vi "JSON Array To LV Enum.vi"(7 "Name Override":string, 8 "Error In":errorcluster, 10 "JSON Array":string, 11 "Enum Dest Dir":path) -> (0 "Error Out":errorcluster)   [LabVIEW 2011, in "LMH-Toolbox.lvlib" / "LMH-Scripting.lvlib"]
doc: "Script a typedef enum control from a JSON array."
uses:
  LMH-Scripting.lvlib
  <vilib>/Utility/miscctls.llb/LVPointTypeDef.ctl
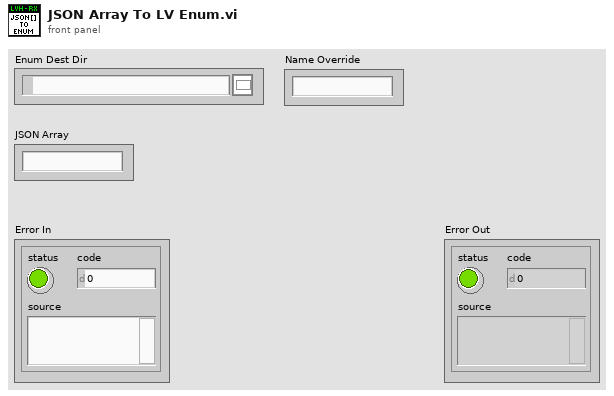
[diagram p1: front panel]
types:
  T1 = enum32{"not a control VI", "control", "typedef", "strict typedef"}
  T2 = typedef "LVPointTypeDef.ctl" = cluster{"Horizontal":i16, "Vertical":i16}
  T3 = enum32{"invalid VI type", "Standard VI", "Control VI", "Global VI", "Polymorphic VI", "Configuration VI", "SubSystem", "Facade VI", "Method VI", "Statechart Diagram VI"}
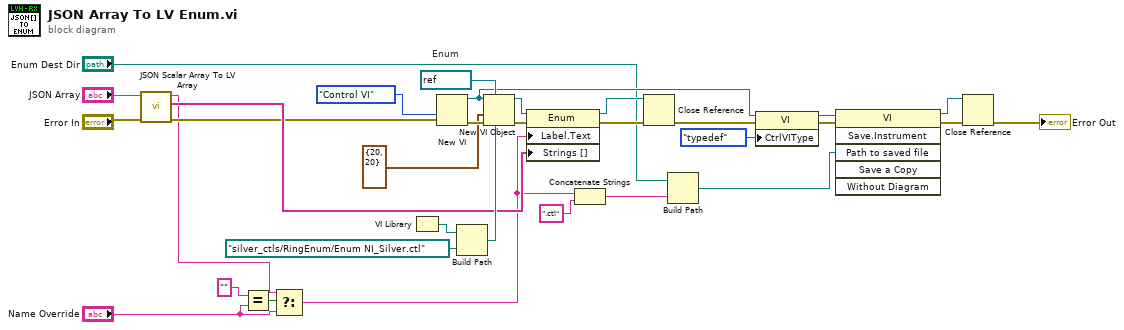
[diagram p0: block diagram]
diagram:
  w31 = refnum<vi> refnum  # Enum
  n1 = call "JSON Scalar Array To LV Array.vi"("Error In"="Error In", "JSON Array"="JSON Array") -> ("Error Out"=w10:errorcluster, "Array Data"=w21:string[], "Array Name"=w2:string)  [unwired: 7 in]
  n2 = Equal?(x="" ("y"), y="Name Override") -> (x = y?=w4:bool)
  n3 = Select(t=w2, s=w4, f="Name Override") -> (s? t:f=w1:string)
  n4 = VI Library() -> (path=w23:path)
  n5 = New VI(8:w10, 9:T3."Control VI" ("vi type (standard vi)")) -> (0:w30:errorcluster, 3:w18:refnum<vi>)  [unwired: 5 in]
  n6 = Build Path(base path=w23, name or relative path=path "silver_ctls/RingEnum/Enum NI_Silver.ctl" ("path")) -> (appended path=w24:path)
  n7 = New VI Object(vi object class=w31, owner refnum=w18, position/next to=T2 {"Horizontal"=20, "Vertical"=20} ("location"), 6:w24, 8:w30) -> (object refnum=w29:refnum<vi>, 0:w28:errorcluster)  [unwired: 3 in]
  n8 = property class="Enum"(reference=w29, error in=w28, "Label.Text"=w1, "Strings []"=w21) -> (reference out=w27:refnum<vi>, error out=w26:errorcluster)
  n9 = Concatenate Strings(w1, ".ctl" ("string")) -> (w8:string)
  n10 = Close Reference(reference=w27, error in (no error)=w26) -> (error out=w19:errorcluster)
  n11 = Build Path(base path="Enum Dest Dir", name or relative path=w8) -> (appended path=w6:path)
  n12 = property class="VI"(reference=w18, error in=w19, "CtrlVIType"=T1."typedef" ("Control VI Type")) -> (reference out=w17:refnum<vi>, error out=w16:errorcluster)
  n13 = invoke class="VI" method="Save.Instrument"(reference=w17, error in=w16, "Path to saved file"=w6) -> (reference out=w15:refnum<vi>, error out=w14:errorcluster)  [unwired: 3 in, 4 out]
  n14 = Close Reference(reference=w15, error in (no error)=w14) -> (error out=→"Error Out":errorcluster)
